vi "Untitled 2222.vi"() -> ()   [LabVIEW 2013]
uses:
  <vilib>/httpClient/POSTBuffer.vi
  <vilib>/httpClient/LabVIEWHTTPClient.lvlib
panel:
  out "error out 2":errorcluster
  out "body 4":string
  out "body 2":string
  out "headers 2":string="HTTP/1.1 200 OK\r\nAppid: 11084351\r\nConnection: keep-alive\r\nContent-Type: application/json\r\nDate: Fri, 13 Apr 2018 09:30:01 GMT\r\nP3p: CP=\" OTI DSP COR IVA OUR IND COM \"\r\nP3p: CP=\" OTI DSP COR IVA OUR IND COM \"\r\nServer: Apache\r\nSet-Cookie: BAIDUID=1F89B6E69B7BBB5C1B4FDF9B6B84EC85:FG=1; expires=Thu, 31-Dec-37 23:55:55 GMT; max-age=2145916555; path=/; domain=.baidu.com; version=1\r\nSet-Cookie: BAIDUID=367536C25070C4B91C130C04903B40D7:FG=1; expires=Thu, 31-Dec-37 23:55:55 GMT; max-age=2145916555; path=/; domain=.baidu.com; version=1\r\nVary: Accept-Encoding\r\nVary: Accept-Encoding\r\nContent-Length: 91\r\n\r\n"
  out "concatenated string 2":string
  in  "Loops":i32=1000
  out "error out":errorcluster
  in  "user":string="charles"
  in  "TEXT(UTF-8)":string
  in  "POST":bool
  out "headers":string
  out "body":string
  out "Numeric":i32
  in  "CN?":bool
  out "Tok 2":string
  out "ok?":bool
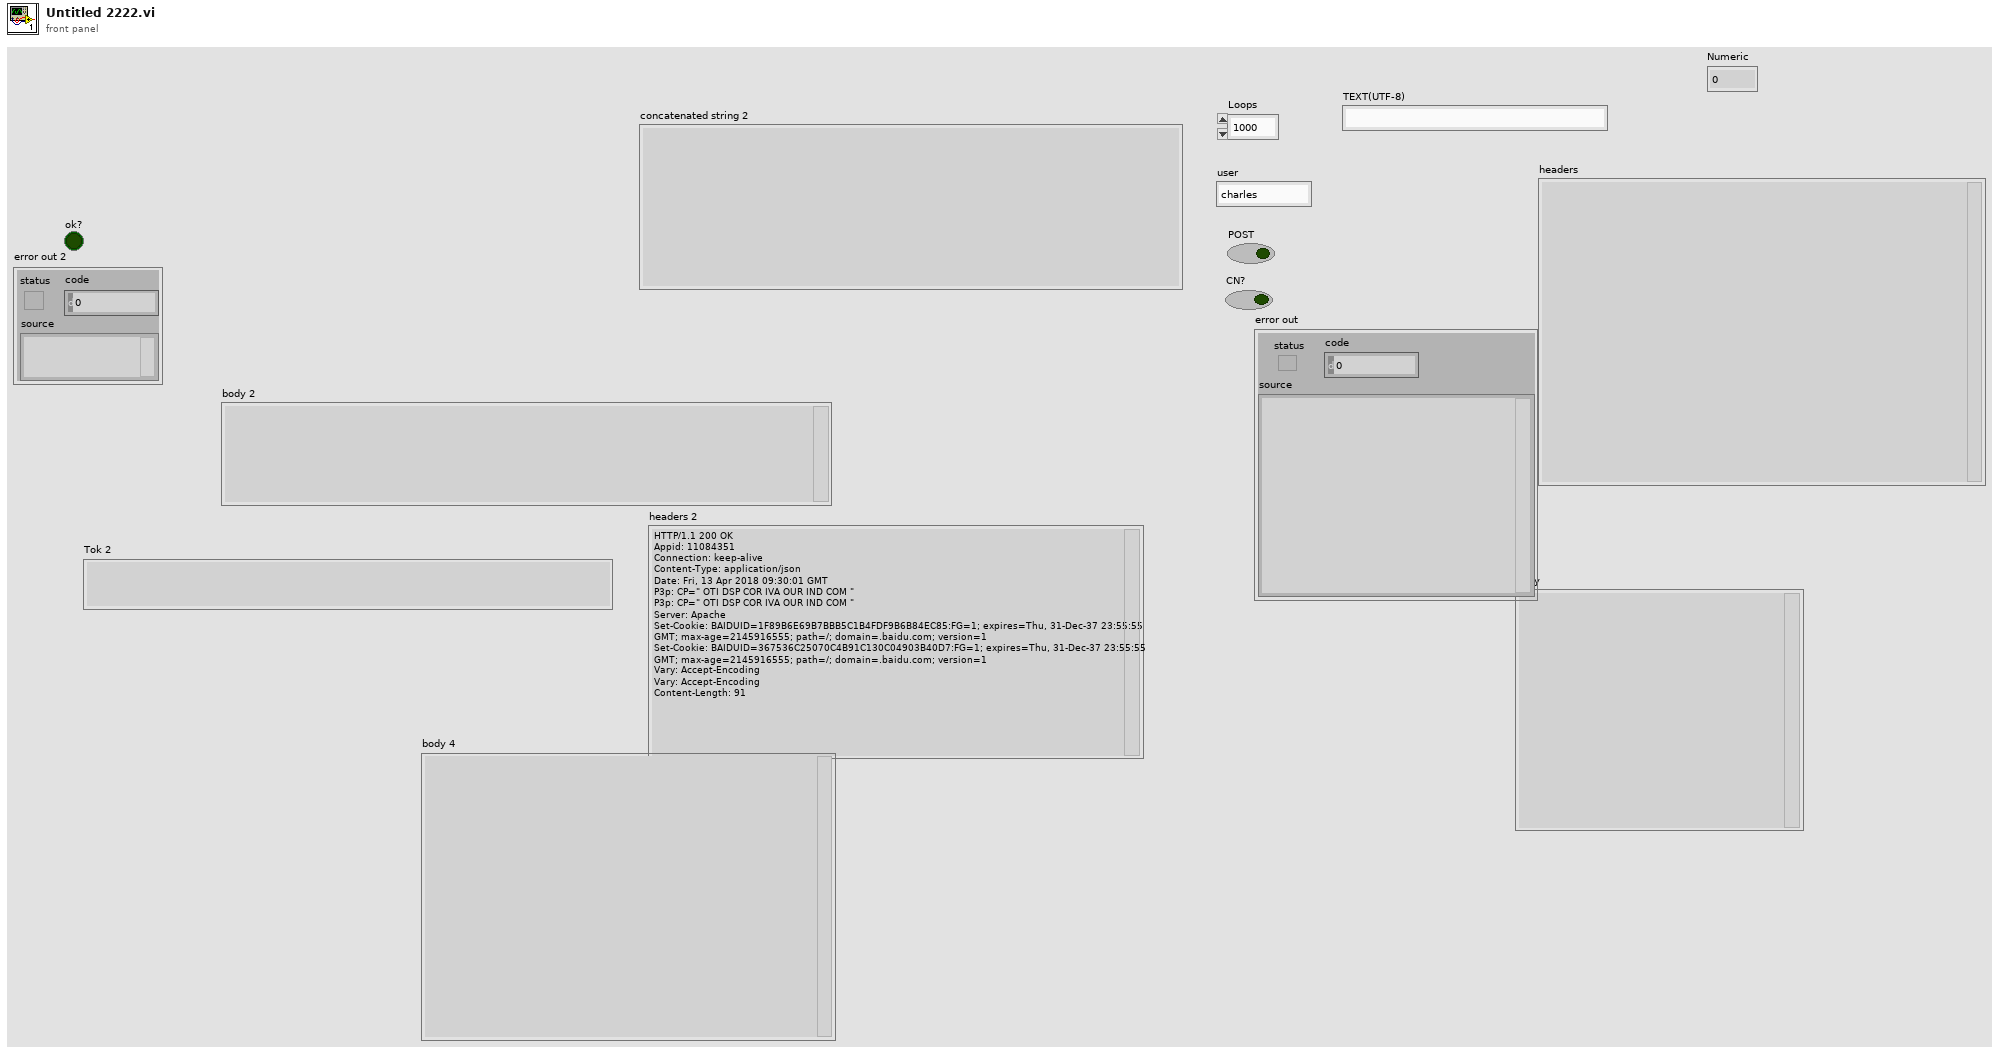
[diagram p1: front panel]
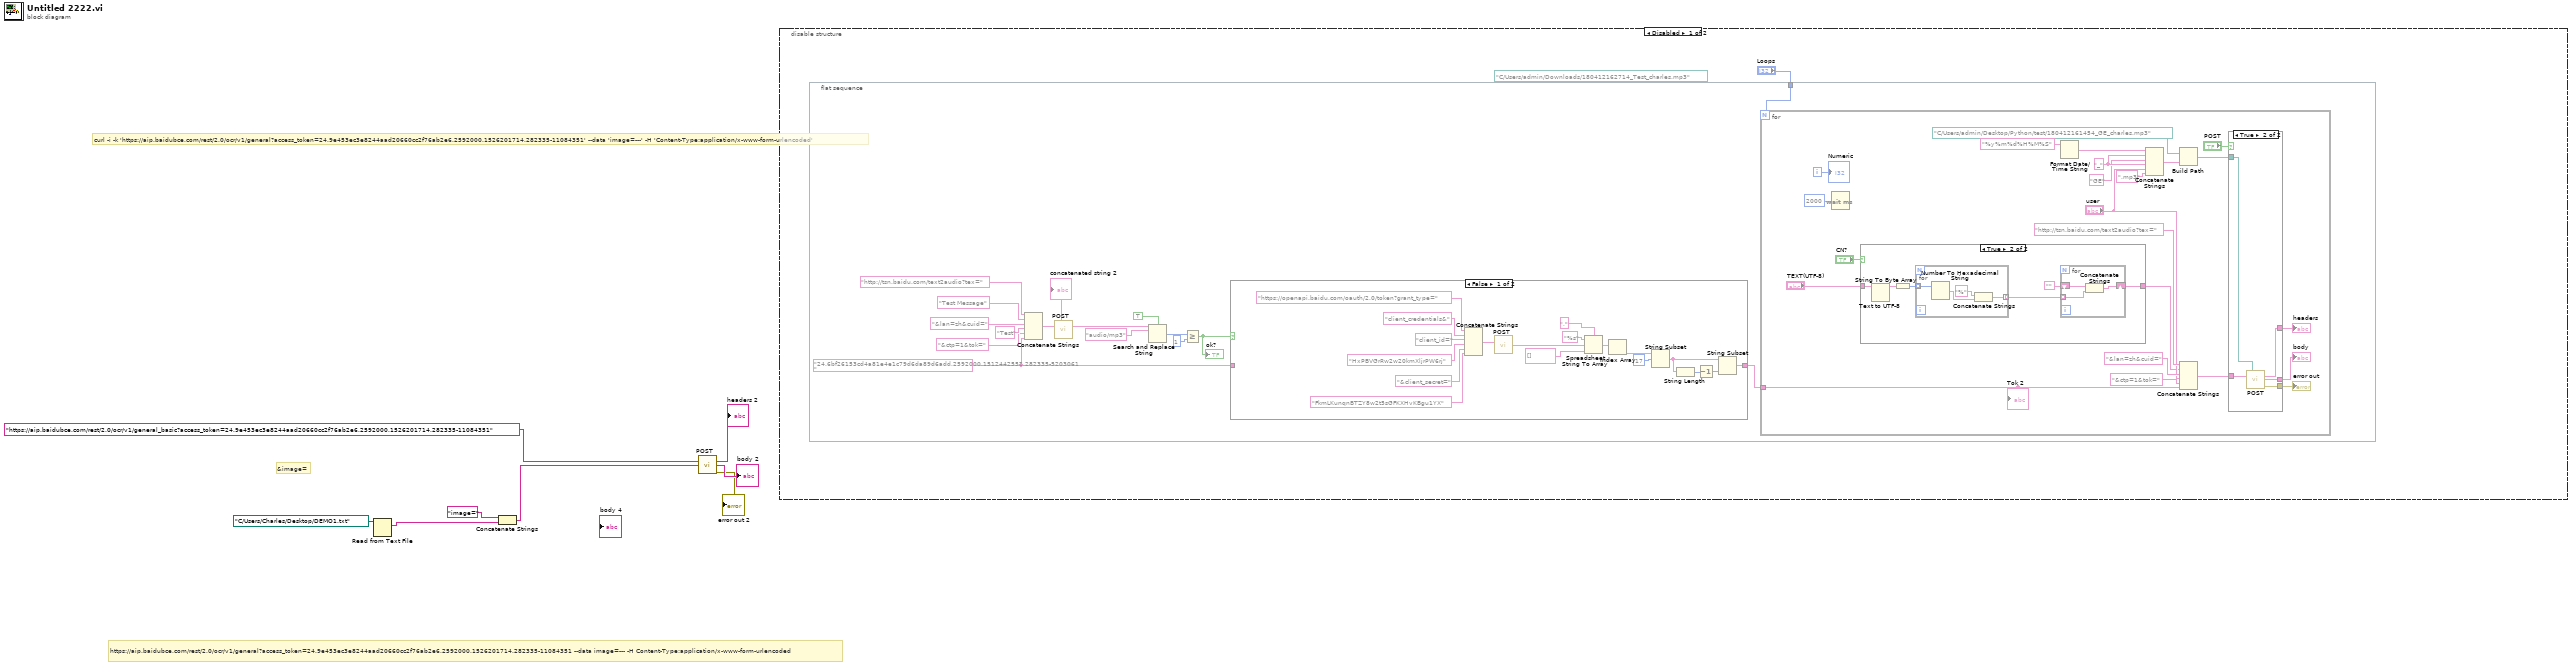
[diagram p0: block diagram]
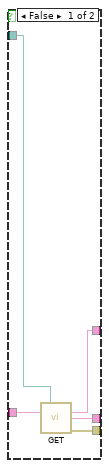
[diagram p4: hidden frame]
diagram:
  # "&image="
  # "https://aip.baidubce.com/rest/2.0/ocr/v1/general?access_token=24.9e453ec3e8244aad20660cc2f76ab2e6.2592000.1526201714.282335-11084351 --data image=--- -H Content-Type:application/x-www-form-urlencoded"
  # "curl -i -k 'https://aip.baidubce.com/rest/2.0/ocr/v1/general?access_token=24.9e453ec3e8244aad20660cc2f76ab2e6.2592000.1526201714.282335-11084351' --data 'image=---' -H 'Content-Type:application/x-www-form-urlencoded'"
  n1 = Read from Text File(file (use dialog)=path "C:/Users/Charles/Desktop/DEMO1.txt") -> (text=w3:string)  [unwired: 3 in, 3 out]
  n2 = Concatenate Strings("image=" ("string"), w3) -> (w1:string)
  n3 = call-poly <vilib>:"POST.vi"("url"="https://aip.baidubce.com/rest/2.0/ocr/v1/general_basic?access_token=24.9e453ec3e8244aad20660cc2f76ab2e6.2592000.1526201714.282335-11084351" ("string"), "buffer"=w1) -> ("headers"=→"headers 2":string, "body"=→"body 2":string, "error out"=→"error out 2":errorcluster)  [unwired: 10 in, 1 out]
  n4 = disable-structure shown="Disabled" {
    frame Disabled {
      (unwired) path "C:/Users/admin/Downloads/180412162714_Test_charles.mp3"
      n5 = flat-sequence {
        tunnel: "Loops" -> [w10]
        frame #0 {
          w12 = "24.6bf26153cd4a81e4e1c79d6da89d6add.2592000.1512442552.282335-5203061" ("Tok 2")
          n6 = Concatenate Strings("http://tsn.baidu.com/text2audio?tex=" ("string"), "Test Message" ("TEXT(UTF-8) 2"), "&lan=zh&cuid=" ("string"), "Test" ("user 2"), "&ctp=1&tok=" ("string"), w12) -> (w21:string)
          "concatenated string 2" <- w21
          n7 = call-poly <vilib>:"POST.vi"("url"=w21) -> ("headers"=w14:string)  [unwired: 11 in, 3 out]
          n8 = Search and Replace String(case sensitive?=TRUE ("ignore case? (F)"), input string=w14, search string="audio/mp3") -> (number of replacements=w16:i32)  [unwired: 5 in, 3 out]
          n9 = Greater Or Equal?(x=w16, y=1) -> (x >= y?=w13:bool)
          "ok?" <- w13
          n10 = case shown="False" w13 {
            tunnel: w12 -> [_ w43]
            tunnel: [w25 w43] -> w11
            frame False {
              n11 = Concatenate Strings("https://openapi.baidu.com/oauth/2.0/token?grant_type=" ("string"), "client_credentials&" ("string"), "client_id=" ("string"), "HxPBVGrRw2w20kmXljrPW6rj" ("string"), "&client_secret=" ("string"), "FkmLKunqnBTZY8w2t5sGFKXHvKBgu1YX" ("string")) -> (w42:string)
              n12 = call-poly <vilib>:"POST.vi"("url"=w42) -> ("body"=w26:string)  [unwired: 11 in, 3 out]
              n13 = Spreadsheet String To Array(delimiter (Tab)=",", format string="%s", spreadsheet string=w26, array type (2D Dbl)=string[] []) -> (array=w32:string[])
              n14 = Index Array(array=w32) -> (element=w31:string)  [unwired: 1 in]
              n15 = String Subset(string=w31, offset (0)=17) -> (substring=w29:string)  [unwired: 1 in]
              n16 = String Length(string=w29) -> (length=w28:i32)
              n17 = Decrement(x=w28) -> (x-1=w27:i32)
              n18 = String Subset(string=w29, length (rest)=w27) -> (substring=w25:string)  [unwired: 1 in]
            }
            frame True {
            }
          }
          n19 = for {
            N: w10 -> [_]
            tunnel: w11 -> [w61]
            i -> [w47]
            w55 = "_" ("string")
            n20 = Wait (ms)(milliseconds to wait=u32 2000) -> ()  [unwired: 1 out]
            n21 = case shown="True" "CN?" {
              tunnel: [w67 w69] -> w46
              tunnel: "TEXT(UTF-8)" -> [w67 w68]
              frame False {
              }
              frame True {
                n22 = Text to UTF-8(11:w68) -> (3:w73:string)  [unwired: 1 in, 1 out]
                n23 = String To Byte Array(string=w73) -> (unsigned byte array=w72:u8[])
                n24 = for {
                  tunnel: w72 -> [w80] mode=indexing
                  tunnel: [w77] -> w71 mode=indexing
                  n25 = Number To Hexadecimal String(2:w80) -> (0:w79:string)  [unwired: 1 in]
                  n26 = Concatenate Strings("%" ("string"), w79) -> (w77:string)
                }
                n27 = for {
                  tunnel: w71 -> [w74] mode=indexing
                  shift-right: [w76] -> w69
                  shift-left: "" -> [w75]
                  n28 = Concatenate Strings(w75, w74) -> (w76:string)
                }
              }
            }
            n29 = Format Date/Time String(time format string (%c)="%y%m%d%H%M%S") -> (date/time string=w53:string)  [unwired: 2 in]
            n30 = Concatenate Strings(w53, w55, "GE" ("string"), w55, "user", ".mp3" ("string")) -> (w58:string)
            n31 = Build Path(base path=path "C:/Users/admin/Desktop/Python/test/180412161454_GE_charles.mp3" ("file (use dialog)"), name or relative path=w58) -> (appended path=w59:path)
            n32 = Concatenate Strings("http://tsn.baidu.com/text2audio?tex=" ("string"), w46, "&lan=zh&cuid=" ("string"), "user", "&ctp=1&tok=" ("string"), w61) -> (w64:string)
            n33 = case shown="True" "POST" {
              tunnel: w64 -> [w84 w90]
              tunnel: [w83 w89] -> w62
              tunnel: w59 -> [w85 w88]
              tunnel: [w82 w87] -> w51
              tunnel: [w81 w86] -> w50
              frame False {
                n34 = call <vilib>:"GET.vi"("output file"=w85, "url"=w84) -> ("headers"=w82:string, "body"=w81:string, "error out"=w83:errorcluster)  [unwired: 10 in, 1 out]
              }
              frame True {
                n35 = call-poly <vilib>:"POST.vi"("output file"=w88, "url"=w90) -> ("headers"=w87:string, "body"=w86:string, "error out"=w89:errorcluster)  [unwired: 10 in, 1 out]
              }
            }
            "error out" <- w62
            "headers" <- w51
            "body" <- w50
            "Numeric" <- w47
            "Tok 2" <- w61
          }
        }
      }
    }
    frame Enabled {
    }
  }
